vi "mmW Reply.vi"(0 "reference in":refnum<class "ZMQ_mmWave.lvclass">, 5 "Multipart message":string[](array[string]), 11 "error in (no error)":errorcluster) -> (4 "reference out":refnum<class "ZMQ_mmWave.lvclass">, 15 "error out":errorcluster)   [LabVIEW 2019, in "CommandResponse communication.lvlib" / "ZMQ_mmWave.lvclass"]
doc: "Replies to previously recieved command with status, info and data"
uses:
  ZMQ_mmWave.lvclass
  C:/Barkhausen mmWave radar/Development/modules/mmw_instrument/src_LabVIEW/Host/Intertarget communication/ZMQ_slave_class/ZMQ_slave.lvclass
  mmw_command_lib/src_LabVIEW/mmW_commands/TypeDefs/response status.ctl
  mmw_command_lib/src_LabVIEW/mmW_commands/commands/typedefs/datatypes_.ctl
  mmw_command_lib/src_LabVIEW/mmW_commands/TypeDefs/commands.ctl
  Host/Intertarget communication/ZMQ_slave_class/ZMQ_slave.lvclass
  <vilib>/addons/zeromq/zmq_socket.lvclass
  Host/Intertarget communication/CommandResponse communication.lvlib
  mmw_command_lib/src_LabVIEW/mmW_commands/mmW_commands.lvlib
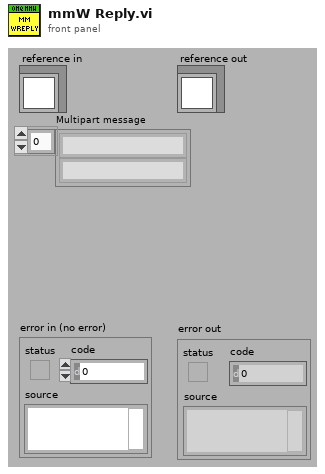
[diagram p1: front panel]
types:
  T1 = typedef "CommandResponse communication.lvlib/ZMQ_slave.lvclass/ObjectAttributes.ctl" = cluster{"ZMQ context":refnum<class "zmq_context.lvclass">, "ZMQ socket":refnum<class "zmq_socket.lvclass">, "endpoint":string}
  T2 = typedef "mmW_commands.lvlib/commands.ctl" = enum16{"configure_fs", "configure_rf", "configure_trigger", "equalization_enable", "equalization_start", "lo_sync_enable", "equalization_stop", "get_instrument_status", "get_versions", "initialize_hw", "pop_rx", "set_log_level", "Shutdown", "start", "start_instrument_app", "stop", "trans", "transceive", "trigger_burst", "trigger_sync_enable", "Write TX", "resp_generic", "resp_waveform", "send_trigger", "fetch", "transceive2"}
  T3 = typedef "mmW_commands.lvlib/datatypes_.ctl" = enum16{"none", "string", "interleaved_I16", "interleaved_I32", "I16_array", "I32_array", "JSONstring"}
  T4 = typedef "mmW_commands.lvlib/response status.ctl" = enum16{"OK", "Error", "Warning", "Unknown"}
  T5 = typedef "CommandResponse communication.lvlib/Error response.ctl" = cluster{"code":i32, "message":string, "source":string}
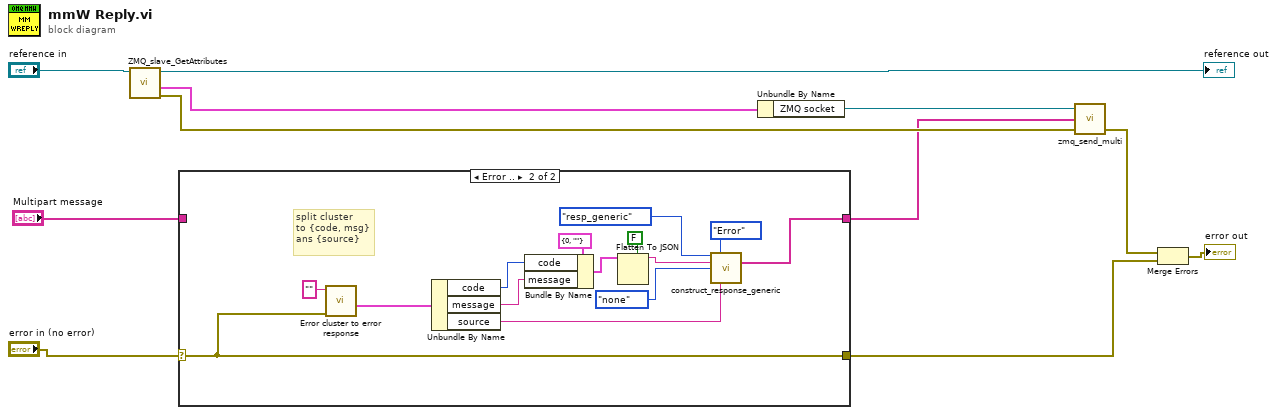
[diagram p0: block diagram]
diagram:
  n1 = call "ZMQ_slave_GetAttributes.vi"("reference in"="reference in") -> ("error out"=w6:errorcluster, "attributes"=w8:T1, "reference out"=→"reference out":refnum<class "ZMQ_mmWave.lvclass">)  [unwired: 7 in, 1 out]
  n2 = case shown="Error .." "error in (no error)" {
    selector: "error in (no error)" -> [_ w26]
    tunnel: [_ w26] -> w3
    tunnel: [w12 w15] -> w2
    tunnel: "Multipart message" -> [w12 _]
    frame No Error {
    }
    frame Error {
      # "split cluster\nto {code, msg}\nans {source}"
      n3 = call "Error cluster to error response.vi"("error in (no error)"=w26, "response"="") -> ("err cluster"=w16:T5)  [unwired: 7 in, 2 out]
      n4 = Unbundle By Name(w16) -> ("code"=w21:i32, "message"=w20:string, "source"=w23:string)
      n5 = Bundle By Name(cluster=cluster{"code":i32, "message":string} {"code"=0, "message"=""} ("Error response"), "code"=w21, "message"=w20) -> (w19:cluster{"code":i32, "message":string})
      n6 = Flatten To JSON(enable LabVIEW extensions? (T)=FALSE, anything=w19) -> (JSON string=w18:string)  [unwired: 1 in, 1 out]
      n7 = call "construct_response_generic.vi"("command in"=commands."resp_generic", "Status"=response_status."Error", "generic_info"=w18, "datatype"=datatypes_."none", "source"=w23) -> ("Multipart message"=w15:string[])  [unwired: 7 in, 3 out]
    }
  }
  n8 = Unbundle By Name(w8) -> ("ZMQ socket"=w7:refnum<class "zmq_socket.lvclass">)
  n9 = call <vilib>:"zmq_send_multi.vi"("error in"=w6, "parts"=w2, "socket in"=w7) -> ("error out"=w11:errorcluster)  [unwired: 1 in, 1 out]
  n10 = Merge Errors(w11, w3) -> (→"error out":errorcluster)
